vi "Terminate Automation.vi"(8 "error in":errorcluster, 11 "Fault Handler in":refnum<class "Fault Handler.lvclass">) -> (0 "error out":errorcluster, 3 "Fault Handler out":refnum<class "Fault Handler.lvclass">)   [LabVIEW 2023, in "Fault Handler.lvlib" / "Fault Handler.lvclass"]
doc: "This routine can only be called when an error is active, automation is running, and the fault monitor has a reference to the automated software sequence context. \n\nIf all these conditions are met, the software transmits a terminate execution command to the automated software."
uses:
  Library/Fault Handler.lvclass
  Library/Fault Handler.lvclass/Fault Handler.ctl
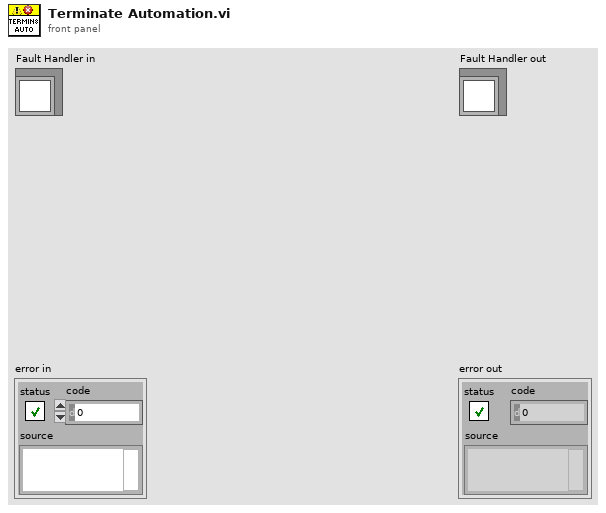
[diagram p1: front panel]
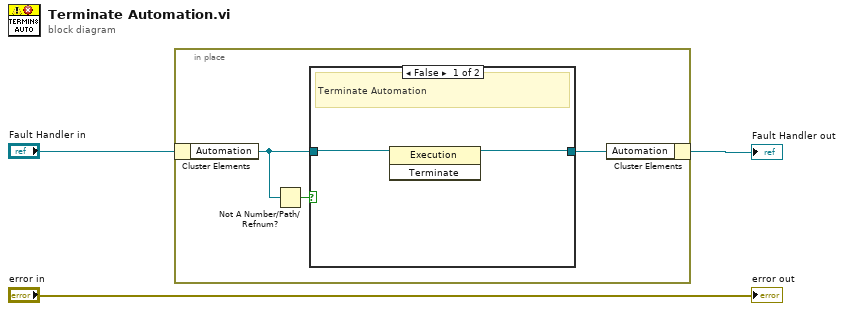
[diagram p0: block diagram]
diagram:
  n1 = in-place {
    n2 = in-place-cluster #1("Fault Handler in") -> ("Automation"=w5:refnum<k7>)
    n3 = Not A Number/Path/Refnum?(number/path/refnum=w5) -> (NaN/Path/Refnum?=w6:bool)
    n4 = case shown="False" w6 {
      tunnel: w5 -> [w8 w9]
      tunnel: [w7 w9] -> w4
      frame False {
        # "Terminate Automation"
        n5 = invoke class="Execution" method="Terminate"(reference=w8) -> (reference out=w7:refnum<k7>)  [unwired: 2 in, 2 out]
      }
      frame True {
        # "Automation Not Running, Ignore"
      }
    }
    n6 = in-place-cluster #1("Automation"=w4) -> (→"Fault Handler out":refnum<class "Fault Handler.lvclass">)
  }
  "error out" <- "error in"
